vi "Alarms.CacheCurrentValues.vi"(8 "error in (no error)":errorcluster, 11 "ListBox in":refnum<vi>) -> (0 "error out":errorcluster, 3 "Alarms":T1[](array[typedef]) {"Delay" format="%.2f"; "Low Limit" format="%.2f"; "High Limit" format="%.2f"})   [LabVIEW 2015, in "Single Station Execution.lvlib"]
uses:
  Single Station Execution.lvlib
  Types/Config.AlarmSettings.ctl
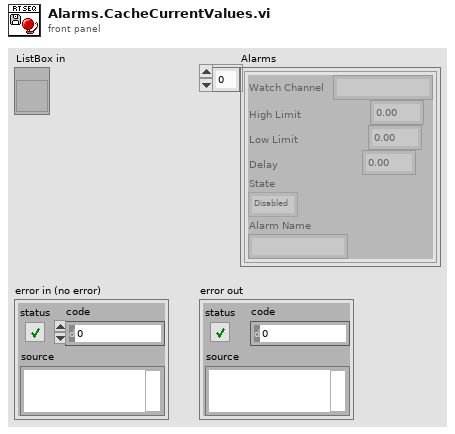
[diagram p1: front panel]
types:
  T1 = typedef "Single Station Execution.lvlib/Config.AlarmSettings.ctl" = cluster{"Watch Channel":string, "High Limit":dbl, "Low Limit":dbl, "Delay":dbl, "State":enum16{"Disabled", "Enabled", "Tripped", "Delayed Trip", "Indicate"}, "Alarm Name":string}
  T2 = enum16{"Disabled", "Enabled", "Tripped", "Delayed Trip", "Indicate"}
  T3 = typedef "NI_VS Alarm ExecutionAPI.lvlib/AlarmInfo.ctl" = cluster{"Watch Channel":string, "High Limit Constant":bool, "High Limit Channel":string, "High Limit":dbl, "Low Limit Constant":bool, "Low Limit Channel":string, "Low Limit":dbl, "Procedure Name":string, "Delay":dbl, "Trip Value":dbl, "Priority":enum16{"Low", "Medium", "High"}, "State":enum16{"Disabled", "Enabled", "Tripped", "Delayed Trip", "Indicate"}, "Mode":enum16{"Normal", "Indicate Only"}, "Group Number":u32, "Priority Number":u32, "Name":string, "Full Name":string}
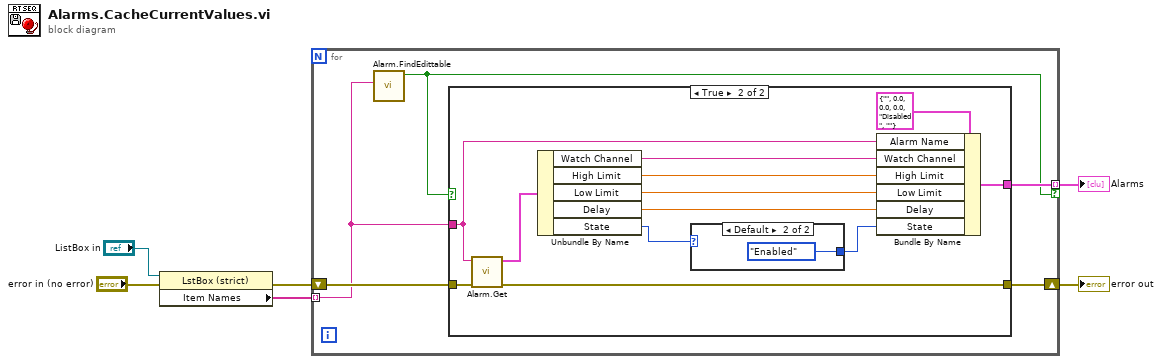
[diagram p0: block diagram]
diagram:
  n1 = property class="LstBox (strict)"(reference="ListBox in", error in="error in (no error)") -> (error out=w4:errorcluster, "Item Names"=w3:string[])  [unwired: 1 out]
  n2 = for {
    tunnel: w3 -> [w8] mode=indexing
    shift-right: [w10] -> w5
    shift-left: w4 -> [w11]
    tunnel: [w9] -> w6 mode=indexing if=w7
    n3 = call "Alarm.FindEdittable.vi"("String"=w8) -> ("Edit?"=w7:bool)  [unwired: 10 in]
    n4 = case shown="True" w7 {
      tunnel: w11 -> [w12 w24]
      tunnel: [w12 w23] -> w10
      tunnel: [_ w16] -> w9
      tunnel: w8 -> [_ w13]
      frame False {
      }
      frame True {
        n5 = call "Alarm.Get.vi"("error in (no error)"=w24, "Alarm"=w13) -> ("error out"=w23:errorcluster, "Alarm Data"=w22:T3)  [unwired: 8 in]
        n6 = Unbundle By Name(w22) -> ("Watch Channel"=w20:string, "High Limit"=w19:dbl, "Low Limit"=w18:dbl, "Delay"=w17:dbl, "State"=w15:T2)
        n7 = case shown="Default" w15 {
          selector: w15 -> [w25 _]
          tunnel: [w25 T2."Enabled" ("State")] -> w14
          frame "Disabled" {
          }
          frame Default {
          }
        }
        n8 = Bundle By Name(cluster=T1 {"Watch Channel"="", "High Limit"=0.0, "Low Limit"=0.0, "Delay"=0.0, "State"=enum."Disabled", "Alarm Name"=""} ("Alarm.Settings"), "Alarm Name"=w13, "Watch Channel"=w20, "High Limit"=w19, "Low Limit"=w18, "Delay"=w17, "State"=w14) -> (w16:T1)
      }
    }
  }
  "Alarms" <- w6
  "error out" <- w5
